vi "test_Timestamp (bad file).vi"(8 "error in (no error)":errorcluster, 11 "TestCase in":refnum<class "Test Read File.lvclass">) -> (0 "error out":errorcluster, 3 "TestCase out":refnum<class "Test Read File.lvclass">)   [LabVIEW 2019, in "Test Read File.lvclass"]
uses:
  Test Read File.lvclass
  C:/Program Files/National Instruments/LabVIEW 2024/vi.lib/Astemes/LUnit/Test Case.lvclass
  <vilib>/Astemes/LUnit/Test Case.lvclass/Test Case.ctl
  11d78fdf-766b-4f18-90a1-9e1853ccfd63.vi
  <vilib>/Astemes/LUnit/Core/LUnit Test Case/Private/Append Fail Result.vi
  <vilib>/Astemes/LUnit/Core/LUnit Test Case/Private/Append Pass Result.vi
  11d78fdf-766b-4f18-90a1-9e1853ccfd63.vi/9c5d11cd-9439-4240-a1ee-d9baace9c924.vi
  <vilib>/Astemes/LUnit/Core/LUnit Test Case/Private/Run In UI.vi
  <vilib>/Utility/error.llb/Clear Errors.vi
  Read/Read Section - Timestamp.vi
  TSC File IO.lvlib
  <vilib>/Astemes/LUnit/Test Case.lvclass
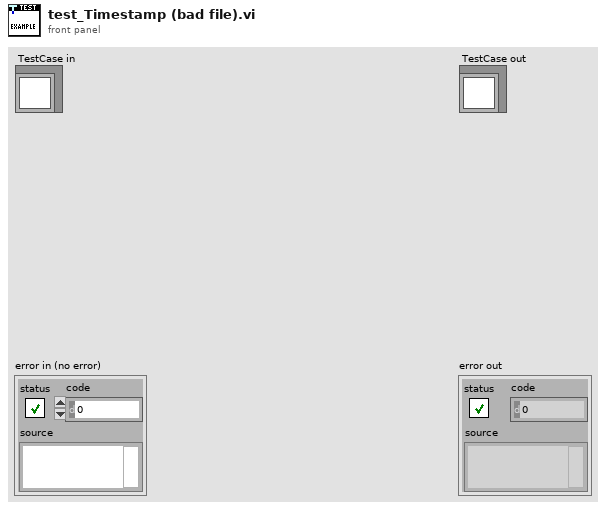
[diagram p1: front panel]
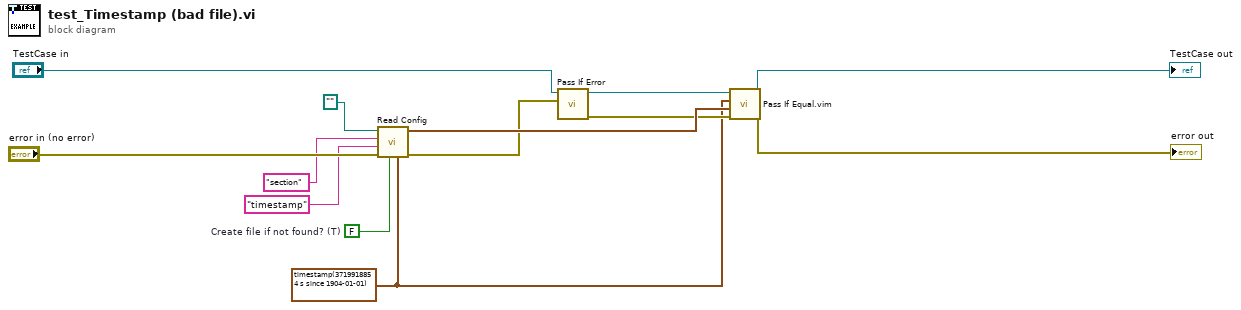
[diagram p0: block diagram]
diagram:
  w2 = timestamp(3719918854.455 s since 1904-01-01) ("Default")
  w7 = FALSE  # Create file if not found? (T)
  n1 = call-poly "Read Config.vi"("Default"=w2, "Create file if not found? (T)"=w7, "error in (no error)"="error in (no error)", "key"="timestamp", "section"="section" ("key"), "Path"=path "") -> ("error out"=w5:errorcluster, "Value"=w9:timestamp)  [unwired: 4 in]
  n2 = call <vilib>:"Pass If Error.vi"("Assert error"=w5, "LUnit Test Case In"="TestCase in") -> ("error out"=w3:errorcluster, "LUnit Test Case Out"=w4:refnum<class "Test Read File.lvclass">)  [unwired: 8 in]
  n3 = call "Pass If Equal.vim"("error in (no error)"=w3, "Actual"=w9, "Expected"=w2, "LUnit Test Case In"=w4) -> ("error out"=→"error out":errorcluster, "LUnit Test Case Out"=→"TestCase out":refnum<class "Test Read File.lvclass">)  [unwired: 6 in]
